vi "complete folders.vi"() -> ()   [LabVIEW 2012]
panel:
  in  "error in":errorcluster
  out "error out":errorcluster
  in  "root folder":path
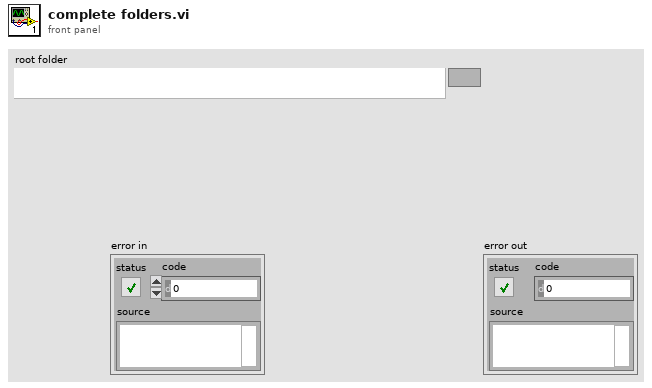
[diagram p1: front panel]
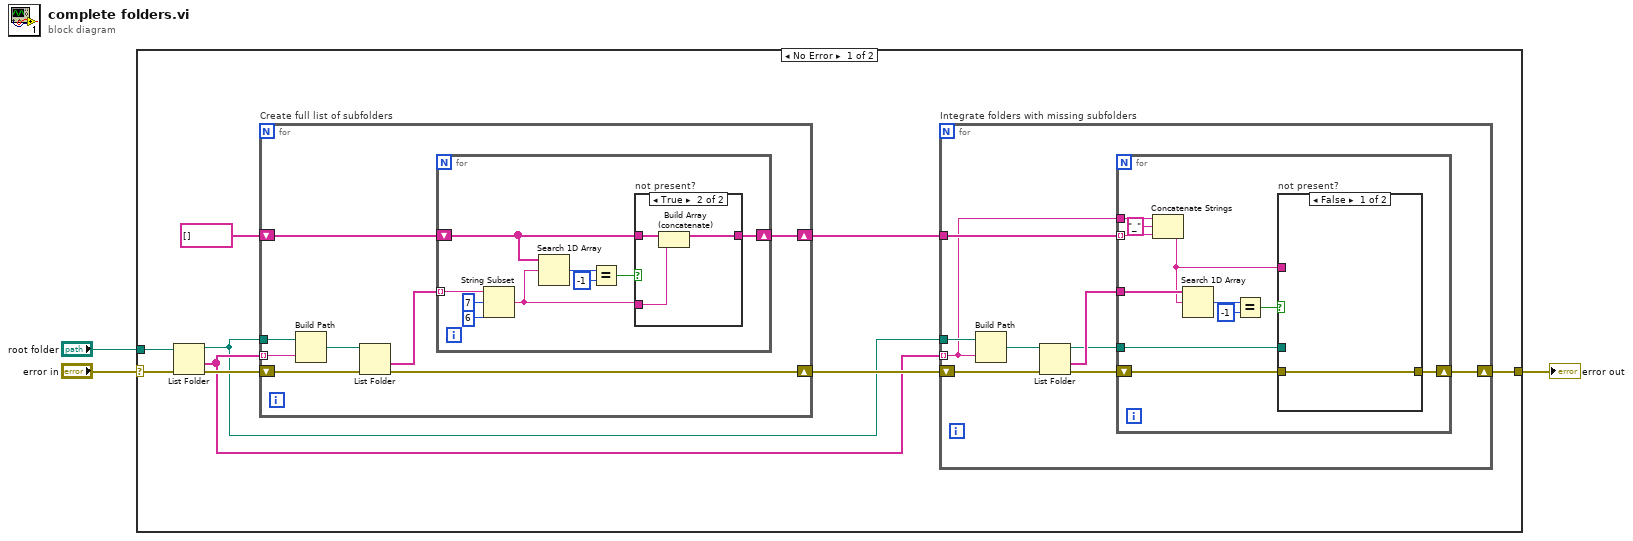
[diagram p0: block diagram]
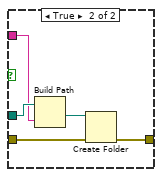
[diagram p2: hidden frame]
diagram:
  n1 = case shown="No Error" "error in" {
    selector: "error in" -> [w4 w60]
    tunnel: "root folder" -> [w12 _]
    tunnel: [w5 w60] -> w2
    frame No Error {
      n2 = List Folder(path=w12, error in=w4) -> (path out=w6:path, folder names=w7:string[], error out=w11:errorcluster)  [unwired: 2 in, 1 out]
      n3 = for "Create full list of subfolders" {
        tunnel: w7 -> [w45] mode=indexing
        tunnel: w6 -> [w46]
        shift-right: [w41] -> w8
        shift-left: w11 -> [w43]
        shift-right: [w39] -> w9
        shift-left: string[] [] ("1D array") -> [w40]
        n4 = Build Path(base path=w46, name or relative path=w45) -> (appended path=w44:path)
        n5 = List Folder(path=w44, error in=w43) -> (folder names=w42:string[], error out=w41:errorcluster)  [unwired: 2 in, 2 out]
        n6 = for {
          tunnel: w42 -> [w55] mode=indexing
          shift-right: [w47] -> w39
          shift-left: w40 -> [w49]
          n7 = String Subset(string=w55, offset (0)=7, length (rest)=6 ("length (rest)")) -> (substring=w48:string)
          n8 = Search 1D Array(1D array=w49, element=w48) -> (index of element=w52:i32)  [unwired: 1 in]
          n9 = Equal?(x=w52, y=-1) -> (x = y?=w50:bool)
          n10 = case "not present?" shown="True" w50 {
            tunnel: w49 -> [w56 w59]
            tunnel: w48 -> [_ w58]
            tunnel: [w56 w57] -> w47
            frame False {
            }
            frame True {
              n11 = Build Array (concatenate)(w59, w58) -> (w57:string[])
            }
          }
        }
      }
      n12 = for "Integrate folders with missing subfolders" {
        tunnel: w7 -> [w16] mode=indexing
        tunnel: w6 -> [w21]
        shift-right: [w14] -> w5
        shift-left: w8 -> [w19]
        tunnel: w9 -> [w17]
        n13 = Build Path(base path=w21, name or relative path=w16) -> (appended path=w20:path)
        n14 = List Folder(path=w20, error in=w19) -> (path out=w13:path, folder names=w18:string[], error out=w15:errorcluster)  [unwired: 2 in, 1 out]
        n15 = for {
          tunnel: w18 -> [w26]
          tunnel: w17 -> [w28] mode=indexing
          tunnel: w16 -> [w29]
          shift-right: [w24] -> w14
          shift-left: w15 -> [w25]
          tunnel: w13 -> [w23]
          n16 = Concatenate Strings(w29, "_" ("string"), w28) -> (w22:string)
          n17 = Search 1D Array(1D array=w26, element=w22) -> (index of element=w32:i32)  [unwired: 1 in]
          n18 = Equal?(x=w32, y=-1) -> (x = y?=w30:bool)
          n19 = case "not present?" shown="False" w30 {
            tunnel: w22 -> [_ w35]
            tunnel: w25 -> [w33 w38]
            tunnel: [w33 w37] -> w24
            tunnel: w23 -> [_ w36]
            frame False {
            }
            frame True {
              n20 = Build Path(base path=w36, name or relative path=w35) -> (appended path=w34:path)
              n21 = Create Folder(path (use dialog)=w34, error in=w38) -> (error out=w37:errorcluster)  [unwired: 1 in, 2 out]
            }
          }
        }
      }
    }
    frame Error {
    }
  }
  "error out" <- w2
